vi "Set Ethernet Physical Layer Configuration.vi"(8 "error in (no error)":errorcluster, 9 "Value":bool, 10 "Configuration (Enable/disable Auto-negotiation of link speed)":i32(ring) items=["Enable/disable Auto-negotiation of link speed", "Set link speed to 10 Base-T or 100 Base T"], 11 "VISA resource name":refnum<visa-resource-name>) -> (0 "error out":errorcluster, 3 "VISA resource name out":refnum<visa-resource-name>, 4 "Device Errors":cluster{"code":i32, "Text":string}[](array[cluster]))   [LabVIEW 2014, in "Stanford Research DG645 - Driver.lvlib"]
doc: "Interface Command: EPHY i,j\nInstrument Error Check\n\nSet the physical configuration item i to j. The parameter i may be one of the following:\n\ni Configuration\n0 Enable Auto-negotiation of link speed?\n1 Set link speed to 10 Base-T or 100 Base-T\n\nIf auto-negotiation is enabled, the manual link speed selection is ignored. When auto negotiation is disabled, the manual speed selection is used to configure the link. Due to a bug in the silicon for the microprocessor, the auto-negotiation of link speed can fail. To avoid this bug, the DG645 defaults to manually configured 100 Base-T link speed.\n\nTo disable Auto-negotiation, set value to false (true otherwise). \n\nTo set 10 Base-T, set value to false (true otherwise)."
uses:
  Stanford Research DG645 - Driver.lvlib
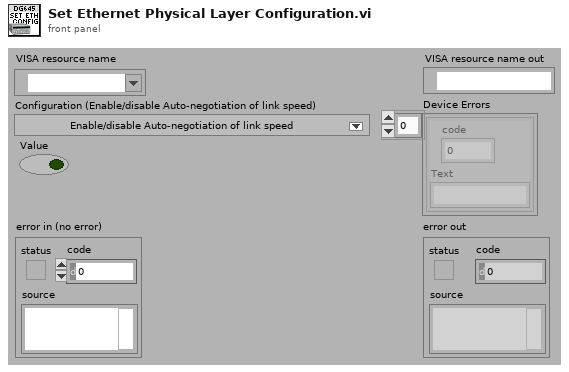
[diagram p1: front panel]
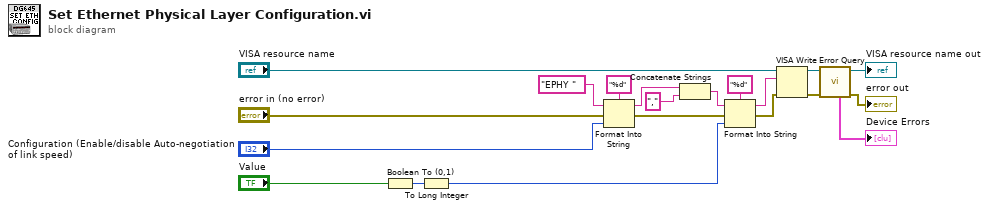
[diagram p0: block diagram]
diagram:
  n1 = Boolean To (0,1)(Boolean="Value") -> (0, 1=w4:i16)
  n2 = To Long Integer(number=w4) -> (32bit integer=w2:i32)
  n3 = Format Into String(format string="%d", initial string="EPHY " ("command"), error in="error in (no error)", "Configuration (Enable/disable Auto-negotiation of link speed)") -> (resulting string=w15:string, error out=w16:errorcluster)
  n4 = Concatenate Strings(w15, "," ("command")) -> (w11:string)
  n5 = Format Into String(format string="%d", initial string=w11, error in=w16, w2) -> (resulting string=w5:string, error out=w6:errorcluster)
  n6 = VISA Write(VISA resource name="VISA resource name", write buffer=w5, error in (no error)=w6) -> (VISA resource name out=w9:refnum<visa-resource-name>, error out=w8:errorcluster)  [unwired: 1 out]
  n7 = call "Error Query.vi"("error in (no error)"=w8, "VISA resource name"=w9) -> ("error out"=→"error out":errorcluster, "VISA resource name out"=→"VISA resource name out":refnum<visa-resource-name>, "Device Errors"=→"Device Errors":cluster{"code":i32, "Text":string}[])  [unwired: 7 in]
